vi "Stoerungs-Queue in Array.vi"(9 "Störmeldetexte aus Datei":string[](array[string]), 11 "Queue-Inhalt (FGV Störmeldungen)":T1[](array[typedef])) -> (3 "Tabelle Störmeldungen":string[](array[string]))   [LabVIEW 2020, in "Stoerungen.lvlib"]
uses:
  Stoerungen.lvlib
  Stoermeldung.ctl
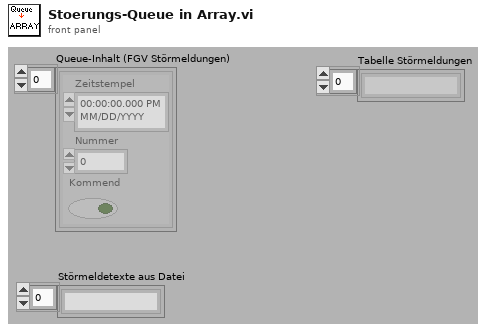
[diagram p1: front panel]
types:
  T1 = typedef "Stoerungen.lvlib/Stoermeldung.ctl" = cluster{"Zeitstempel":timestamp, "Nummer":i32, "Kommend":bool}
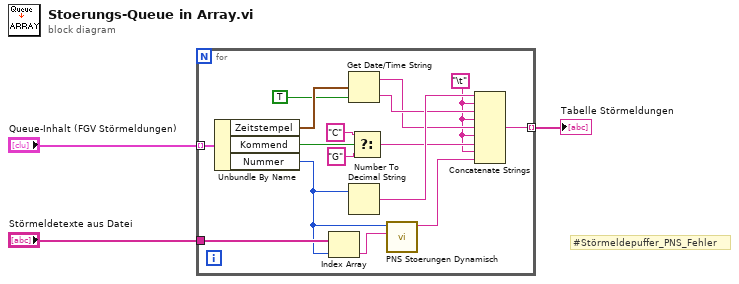
[diagram p0: block diagram]
diagram:
  # "#Störmeldepuffer_PNS_Fehler"
  n1 = for {
    tunnel: "Queue-Inhalt (FGV Störmeldungen)" -> [w19] mode=indexing
    tunnel: "Störmeldetexte aus Datei" -> [w18]
    tunnel: [w7] -> w1 mode=indexing
    w8 = "\t"
    n2 = Unbundle By Name(w19) -> ("Zeitstempel"=w17:timestamp, "Kommend"=w15:bool, "Nummer"=w5:i32)
    n3 = Index Array(array=w18, index=w5) -> (element=w4:string)
    n4 = Get Date/Time String(seconds (now)=w17, want seconds? (F)=TRUE ("Angabe von Sekunden? (F)")) -> (date string=w10:string, time string=w11:string)  [unwired: 1 out]
    n5 = Number To Decimal String(number=w5) -> (decimal integer string=w12:string)  [unwired: 1 out]
    n6 = Select(t="C", s=w15, f="G") -> (s? t:f=w9:string)
    n7 = call "PNS Stoerungen Dynamisch.vi"("Störmeldetexte"=w4, "Nummer"=w5) -> ("String"=w6:string)  [unwired: 9 in]
    n8 = Concatenate Strings(w12, w8, w11, w8, w10, w8, w9, w8, w6) -> (w7:string)
  }
  "Tabelle Störmeldungen" <- w1
